vi "stepper_init.vi"(7 "MG17Motor":refnum<k7>(container), 8 "travel limits":T4={"pfRevPosLimit"=0.0, "pfFwdPosLimit"=4.0, "plLimitMode"=0}, 9 "velocity parameters":T3={"pfMinVel"=0.0, "pfAccn"=4.0, "pfMaxVel"=4.0}, 10 "parameter set":string="dha_apt_stepper", 11 "HWSerialNum":i32=90897058) -> (0 "error out":errorcluster, 1 "travel limits":T2, 2 "velocity parameters":T1, 3 "reference out":refnum<k7>)   [LabVIEW 2018]
uses:
  <userlib>/stepper/travel limits.ctl
  <userlib>/stepper/velocity settings.ctl
panel:
  in  "error in (no error)":errorcluster
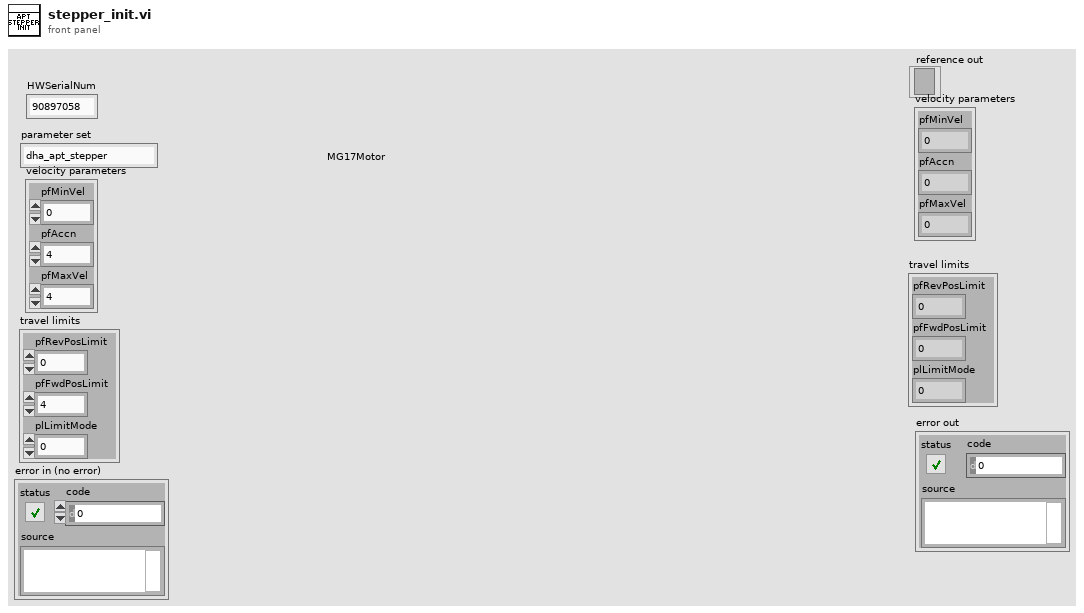
[diagram p1: front panel]
types:
  T1 = cluster{"pfMinVel":sgl, "pfAccn":sgl, "pfMaxVel":sgl}
  T2 = cluster{"pfRevPosLimit":sgl, "pfFwdPosLimit":sgl, "plLimitMode":i32}
  T3 = typedef "velocity settings.ctl" = cluster{"pfMinVel":sgl, "pfAccn":sgl, "pfMaxVel":sgl}
  T4 = typedef "travel limits.ctl" = cluster{"pfRevPosLimit":sgl, "pfFwdPosLimit":sgl, "plLimitMode":i32}
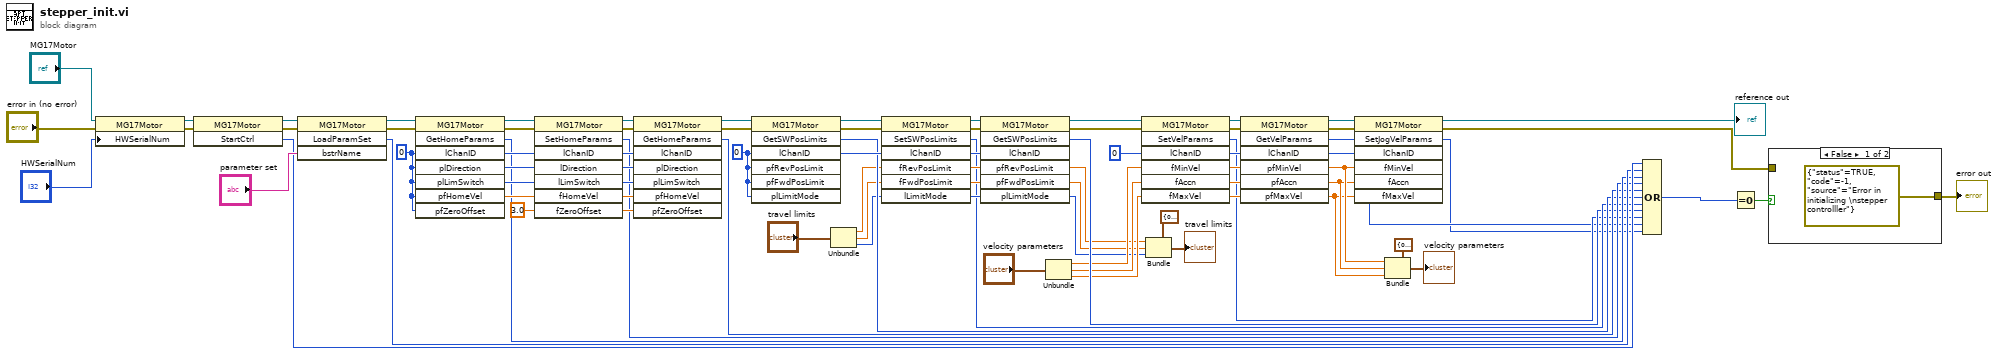
[diagram p0: block diagram]
diagram:
  w32 = 0 ("lChanID")
  w65 = 0 ("lChanID")
  n1 = property class="MG17Motor"(reference="MG17Motor", error in="error in (no error)", "HWSerialNum"="HWSerialNum") -> (reference out=w81:refnum<k7>, error out=w25:errorcluster)
  n2 = invoke class="MG17Motor" method="StartCtrl"(reference=w81, error in=w25) -> (reference out=w80:refnum<k7>, error out=w24:errorcluster, "StartCtrl"=w46:i32)  [unwired: 1 in]
  n3 = invoke class="MG17Motor" method="LoadParamSet"(reference=w80, error in=w24, "bstrName"="parameter set") -> (reference out=w72:refnum<k7>, error out=w23:errorcluster, "LoadParamSet"=w45:i32)  [unwired: 1 in, 1 out]
  n4 = invoke class="MG17Motor" method="GetHomeParams"(reference=w72, error in=w23, "lChanID"=w65, "plDirection"=w65, "plLimSwitch"=w65, "pfHomeVel"=w65, "pfZeroOffset"=w65) -> (reference out=w78:refnum<k7>, error out=w77:errorcluster, "GetHomeParams"=w44:i32, "lChanID"=w76:i32, "plDirection"=w75:i32, "plLimSwitch"=w74:i32, "pfHomeVel"=w73:sgl)  [unwired: 1 in, 1 out]
  n5 = invoke class="MG17Motor" method="SetHomeParams"(reference=w78, error in=w77, "lChanID"=w76, "lDirection"=w75, "lLimSwitch"=w74, "fHomeVel"=w73, "fZeroOffset"=sgl 3.0) -> (reference out=w66:refnum<k7>, error out=w22:errorcluster, "SetHomeParams"=w43:i32, "lChanID"=w67:i32, "lDirection"=w68:i32, "lLimSwitch"=w69:i32, "fHomeVel"=w70:sgl, "fZeroOffset"=w71:sgl)  [unwired: 1 in]
  n6 = invoke class="MG17Motor" method="GetHomeParams"(reference=w66, error in=w22, "lChanID"=w67, "plDirection"=w68, "plLimSwitch"=w69, "pfHomeVel"=w70, "pfZeroOffset"=w71) -> (reference out=w63:refnum<k7>, error out=w21:errorcluster, "GetHomeParams"=w42:i32)  [unwired: 1 in, 5 out]
  n7 = invoke class="MG17Motor" method="GetSWPosLimits"(reference=w63, error in=w21, "lChanID"=w32, "pfRevPosLimit"=w32, "pfFwdPosLimit"=w32, "plLimitMode"=w32) -> (reference out=w62:refnum<k7>, error out=w20:errorcluster, "GetSWPosLimits"=w41:i32, "lChanID"=w61:i32)  [unwired: 1 in, 3 out]
  n8 = Unbundle("travel limits") -> ("pfRevPosLimit"=w33:sgl, "pfFwdPosLimit"=w34:sgl, "plLimitMode"=w35:i32)
  n9 = invoke class="MG17Motor" method="SetSWPosLimits"(reference=w62, error in=w20, "lChanID"=w61, "fRevPosLimit"=w33, "fFwdPosLimit"=w34, "lLimitMode"=w35) -> (reference out=w60:refnum<k7>, error out=w19:errorcluster, "SetSWPosLimits"=w40:i32, "lChanID"=w59:i32, "fRevPosLimit"=w58:sgl, "fFwdPosLimit"=w57:sgl, "lLimitMode"=w56:i32)  [unwired: 1 in]
  n10 = invoke class="MG17Motor" method="GetSWPosLimits"(reference=w60, error in=w19, "lChanID"=w59, "pfRevPosLimit"=w58, "pfFwdPosLimit"=w57, "plLimitMode"=w56) -> (reference out=w55:refnum<k7>, error out=w18:errorcluster, "GetSWPosLimits"=w39:i32, "pfRevPosLimit"=w12:sgl, "pfFwdPosLimit"=w11:sgl, "plLimitMode"=w10:i32)  [unwired: 1 in, 1 out]
  n11 = Unbundle("velocity parameters") -> ("pfMinVel"=w31:sgl, "pfAccn"=w30:sgl, "pfMaxVel"=w29:sgl)
  n12 = invoke class="MG17Motor" method="SetVelParams"(reference=w55, error in=w18, "lChanID"=0, "fMinVel"=w31, "fAccn"=w30, "fMaxVel"=w29) -> (reference out=w53:refnum<k7>, error out=w17:errorcluster, "SetVelParams"=w38:i32, "lChanID"=w52:i32, "fMinVel"=w51:sgl, "fAccn"=w50:sgl, "fMaxVel"=w49:sgl)  [unwired: 1 in]
  n13 = Bundle(cluster=T2 {"pfRevPosLimit"=0.0, "pfFwdPosLimit"=4.0, "plLimitMode"=3} ("travel limits"), "pfRevPosLimit"=w12, "pfFwdPosLimit"=w11, "plLimitMode"=w10) -> (→"travel limits":T2)
  n14 = invoke class="MG17Motor" method="GetVelParams"(reference=w53, error in=w17, "lChanID"=w52, "pfMinVel"=w51, "pfAccn"=w50, "pfMaxVel"=w49) -> (reference out=w48:refnum<k7>, error out=w16:errorcluster, "GetVelParams"=w37:i32, "lChanID"=w47:i32, "pfMinVel"=w8:sgl, "pfAccn"=w7:sgl, "pfMaxVel"=w6:sgl)  [unwired: 1 in]
  n15 = invoke class="MG17Motor" method="SetJogVelParams"(reference=w48, error in=w16, "lChanID"=w47, "fMinVel"=w8, "fAccn"=w7, "fMaxVel"=w6) -> (reference out=→"reference out":refnum<k7>, error out=w1:errorcluster, "SetJogVelParams"=w36:i32)  [unwired: 1 in, 4 out]
  n16 = Bundle(cluster=T1 {"pfMinVel"=0.0, "pfAccn"=4.0, "pfMaxVel"=4.0} ("velocity parameters"), "pfMinVel"=w8, "pfAccn"=w7, "pfMaxVel"=w6) -> (→"velocity parameters":T1)
  n17 = Compound Arithmetic op=OR(w46, w45, w44, w43, w42, w41, w40, w39, w38, w37, w36) -> (w28:i32)
  n18 = Equal To 0?(x=w28) -> (x = 0?=w27:bool)
  n19 = case shown="False" w27 {
    tunnel: [errorcluster {"status"=TRUE, "code"=-1, "source"="Error in initializing \nstepper controlller"} ("error out") w85] -> w15
    tunnel: w1 -> [_ w85]
    frame False {
    }
    frame True {
    }
  }
  "error out" <- w15
